vi "ERRMSGdll.vi"(8 "error in (no error)":errorcluster, 11 "ierr in":i32=1000) -> (0 "error out":errorcluster, 1 "herr_length":i32, 2 "herr":string, 3 "ierr":i32)   [LabVIEW 2015]
doc: "subroutine ERRMSGdll(ierr, herr, herr_length)\n\nRetrieve the last error message saved in calls to ERRNUM (but only if the ierr variable is not equal to zero).\nWrite error messages to default output if iErrPrnt is active. The variable iErrPrnt in the common blocks must\nalways be zero when compiling the DLL.\n\nINPUTS:\nnone\n\nOUTPUTS:\nierr -- Error number from the last call to ERRNUM Output:\nherr -- Associated error string (character*255)\nherr_length -- length of variable herr (default: 255)\n\nOutputs depend on variable iErrPrnt in the common blocks\n• iErrPrnt= 0 - Error string not written (default)\n• iErrPrnt=-1 - Error string written to screen\n• iErrPrnt= 1 - Error string written to screen only if ierr is positive\n• iErrPrnt=3,-3 - Same as 1 and -1, but program also pauses"
uses:
  REFPROP.dll
panel:
  # "REFPROP-ERRMSGdll.vi"
  # "void  ERRMSGdll(int32_t *ierr, CStr herr, int32_t herr_length);"
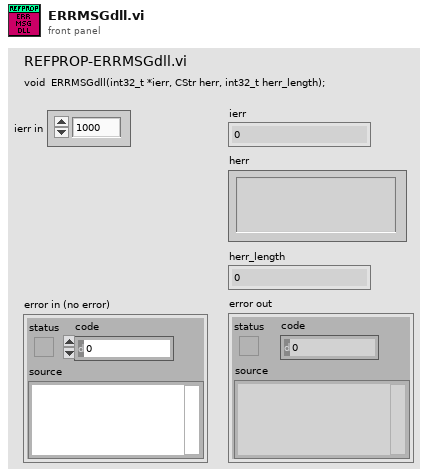
[diagram p1: front panel]
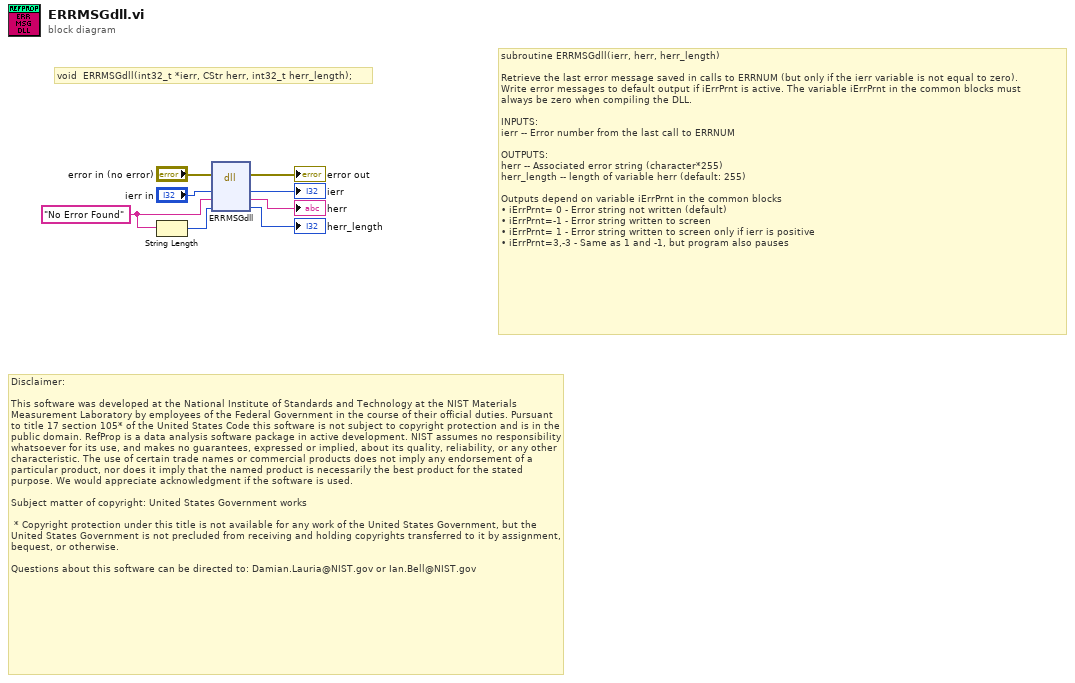
[diagram p0: block diagram]
diagram:
  w4 = "No Error Found"
  # "void  ERRMSGdll(int32_t *ierr, CStr herr, int32_t herr_length);"
  # "Disclaimer:\n\nThis software was developed at the National Institute of Standards and Technology at the NIST Materials Measurement Laboratory by employees of the Federal Government in the course of their official duties. Pursuant to title 17 section 105* of the United States Code this software is not subject to copyright protection and is in the public domain. RefProp is a data analysis software package in active development. NIST assumes no responsibility whatsoever for its use, and makes no guarantees, expressed or implied, about its quality, reliability, or any other characteristic. The use of certain trade names or commercial products does not imply any endorsement of a particular product, nor does it imply that the named product is necessarily the best product for the stated purpose. We would appreciate acknowledgment if the software is used.\n \nSubject matter of copyright: United States Government works\n  \n * Copyright protection under this title is not available for any work of the United States Government, but the United States Government is not precluded from receiving and holding copyrights transferred to it by assignment, bequest, or otherwise.\n\nQuestions about this software can be directed to: Damian.Lauria@NIST.gov or Ian.Bell@NIST.gov"
  # "subroutine ERRMSGdll(ierr, herr, herr_length)\n\nRetrieve the last error message saved in calls to ERRNUM (but only if the ierr variable is not equal to zero).\nWrite error messages to default output if iErrPrnt is active. The variable iErrPrnt in the common blocks must\nalways be zero when compiling the DLL.\n\nINPUTS:\nierr -- Error number from the last call to ERRNUM\n\nOUTPUTS: \nherr -- Associated error string (character*255)\nherr_length -- length of variable herr (default: 255)\n\nOutputs depend on variable iErrPrnt in the common blocks\n• iErrPrnt= 0 - Error string not written (default)\n• iErrPrnt=-1 - Error string written to screen\n• iErrPrnt= 1 - Error string written to screen only if ierr is positive\n• iErrPrnt=3,-3 - Same as 1 and -1, but program also pauses"
  n1 = String Length(string=w4) -> (length=w5:i32)
  n2 = dll-call lib="C:/Users/lauria/Desktop/REFPROP 10 LabVIEW Wrapper BETA/REFPROP/REFPROP.*" fn="ERRMSGdll"(error in="error in (no error)", "ierr"="ierr in", "herr"=w4, "herr_length"=w5) -> (error out=→"error out":errorcluster, "ierr"=→"ierr":i32, "herr"=→"herr":string, "herr_length"=→"herr_length":i32)  [unwired: 3 in, 1 out]
